vi "Read Trigger Settings.vi"(8 "error in (no error)":errorcluster, 11 "AnalogInput in":refnum<class "AnalogInput.lvclass">) -> (0 "error out":errorcluster, 2 "User Trigger Settings":T1={"Timeout"=0.0, "Level"=0.0, "Slope"=enum."Falling", "samples per channel"=100, "Sample Rate (10k)"=10000.0, "pretrigger samples"=500}, 3 "AnalogInput out":refnum<class "AnalogInput.lvclass">)   [LabVIEW 2019, in "AnalogInput.lvlib" / "AnalogInput.lvclass"]
uses:
  Library/AnalogInput.lvclass
  Custom Controls/User Trigger Settings.ctl
  Custom Controls/Trigger_Slope.ctl
  Library/AnalogInput.lvclass/AnalogInput.ctl
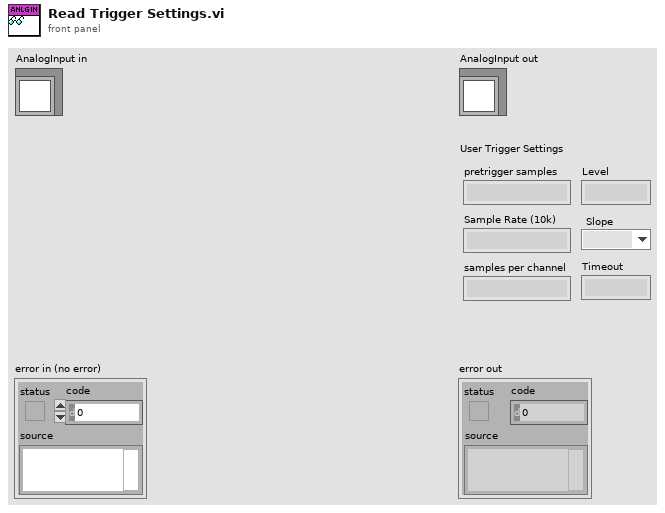
[diagram p1: front panel]
types:
  T1 = typedef "AnalogInput.lvlib/AnalogInput.lvclass/User Trigger Settings.ctl" = cluster{"Timeout":dbl, "Level":dbl, "Slope":T2, "samples per channel":i32, "Sample Rate (10k)":dbl, "pretrigger samples":u32}
  T2 = typedef "AnalogInput.lvlib/AnalogInput.lvclass/Trigger_Slope.ctl" = enum16{"Rising", "Falling"}
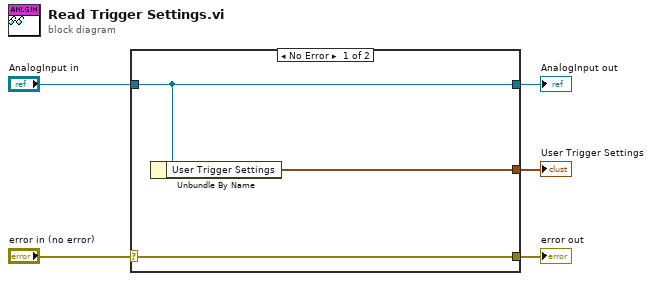
[diagram p0: block diagram]
diagram:
  n1 = case shown="No Error" "error in (no error)" {
    selector: "error in (no error)" -> [w8 w9]
    tunnel: [w8 w9] -> w4
    tunnel: [w7 w10] -> w2
    tunnel: "AnalogInput in" -> [w7 w10]
    tunnel: [w6 _] -> w1
    frame No Error {
      n2 = Unbundle By Name(w7) -> ("User Trigger Settings"=w6:T1)
    }
    frame Error {
    }
  }
  "error out" <- w4
  "AnalogInput out" <- w2
  "User Trigger Settings" <- w1
